vi "State Machine Kernel.vi"(4 "Init?":bool, 5 "Inputs":T4 {"Kobuki Sensors"."Charger Source" items=["DISCHARGING"=0, "DOCKING_CHARGED"=2, "DOCKING_CHARGING"=6, "ADAPTER_CHARGED"=18, "ADAPTER_CHARGING"=22]; "accelerometer"."z axis (g)" format="%.3f"; "accelerometer"."y axis (g)" format="%.3f"; "accelerometer"."x axis (g)" format="%.3f"}, 7 "StateData In":T1) -> (0 "Terminated?":bool, 2 "Outputs":T3, 3 "StateData Out":T1)   [LabVIEW 2017]
uses:
  controls/Inputs.ctl
  shared/Accelerometer.ctl
  Kobuki/KobukiSensors.ctl
  Kobuki/Kobuki Bumps and WheelDrops.ctl
  Kobuki/Kobuki Buttons.ctl
  controls/Outputs.ctl
  controls/StateData.ctl
  controls/StatesEnum.ctl
panel:
  # "Electrical: charging, battery, OI mode"
  # "Sensors: bump, cliff, button, wheel drop"
  # "Motors:"
  # "Inertia"
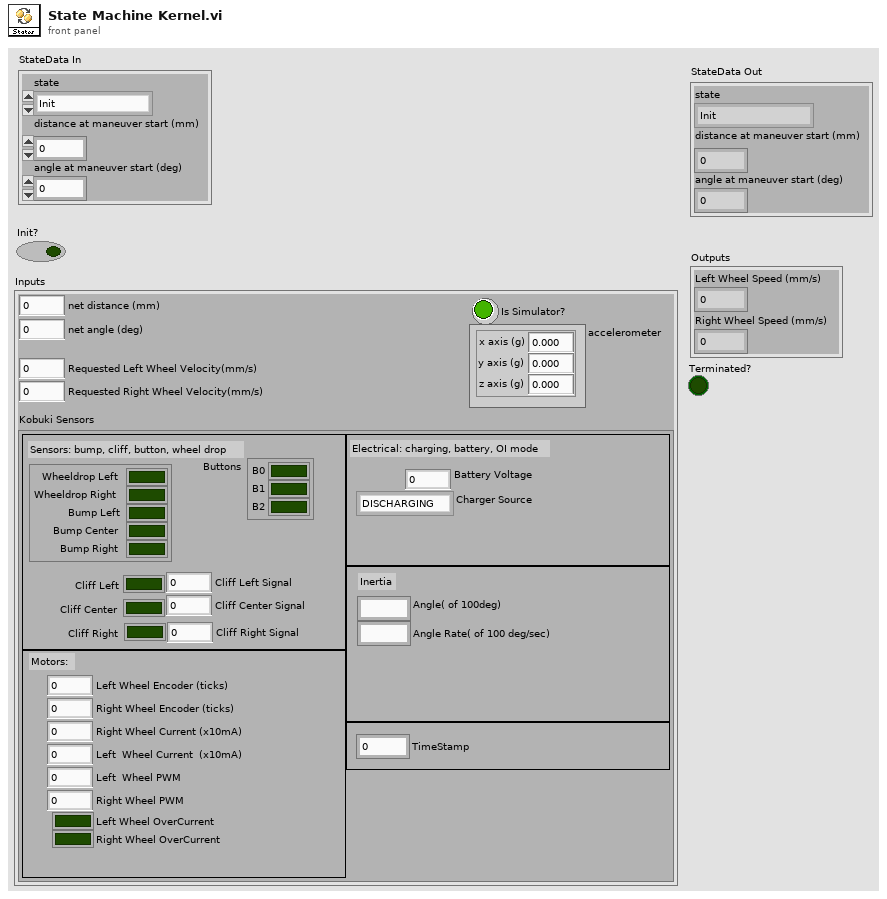
[diagram p1: front panel]
types:
  T1 = typedef "StateData.ctl" = cluster{"distance at maneuver start (mm)":i32, "angle at maneuver start (deg)":i32, "state":T2}
  T2 = typedef "StatesEnum.ctl" = enum16{"Init", "Pause", "Drive", "L.Cliff", "R.Cliff", "Shut"}
  T3 = typedef "Outputs.ctl" = cluster{"Left Wheel Speed (mm/s)":i16, "Right Wheel Speed (mm/s)":i16}
  T4 = typedef "Inputs.ctl" = cluster{"net distance (mm)":i32, "net angle (deg)":i32, "accelerometer":T5, "Is Simulator?":bool, "Kobuki Sensors":T6, "Requested Left Wheel Velocity(mm/s)":i32, "Requested Right Wheel Velocity(mm/s)":i32}
  T5 = typedef "Accelerometer.ctl" = cluster{"x axis (g)":dbl, "y axis (g)":dbl, "z axis (g)":dbl}
  T6 = typedef "KobukiSensors.ctl" = cluster{"Bumps + Wheel Drops":T7, "Cliff Left":bool, "Cliff Center":bool, "Cliff Right":bool, "Cliff Left Signal":u16, "Cliff Center Signal":u16, "Cliff Right Signal":u16, "Buttons":T8, "Left Wheel Encoder (ticks)":u16, "Right Wheel Encoder (ticks) ":u16, "Left  Wheel PWM":i8, "Right Wheel PWM":i8, "Left Wheel OverCurrent":bool, "Right Wheel OverCurrent ":bool, "Right Wheel Current (x10mA)":i16, "Left  Wheel Current  (x10mA)":i16, "TimeStamp":u16, "Battery Voltage":dbl, "Angle( of 100deg)":i16, "Angle Rate( of 100 deg/sec)":i16, "Charger Source ":i8}
  T7 = typedef "Kobuki Bumps and WheelDrops.ctl" = cluster{"Wheeldrop Left":bool, "Wheeldrop Right":bool, "Bump Left":bool, "Bump Center":bool, "Bump Right":bool}
  T8 = typedef "Kobuki Buttons.ctl" = cluster{"B0":bool, "B1":bool, "B2":bool}
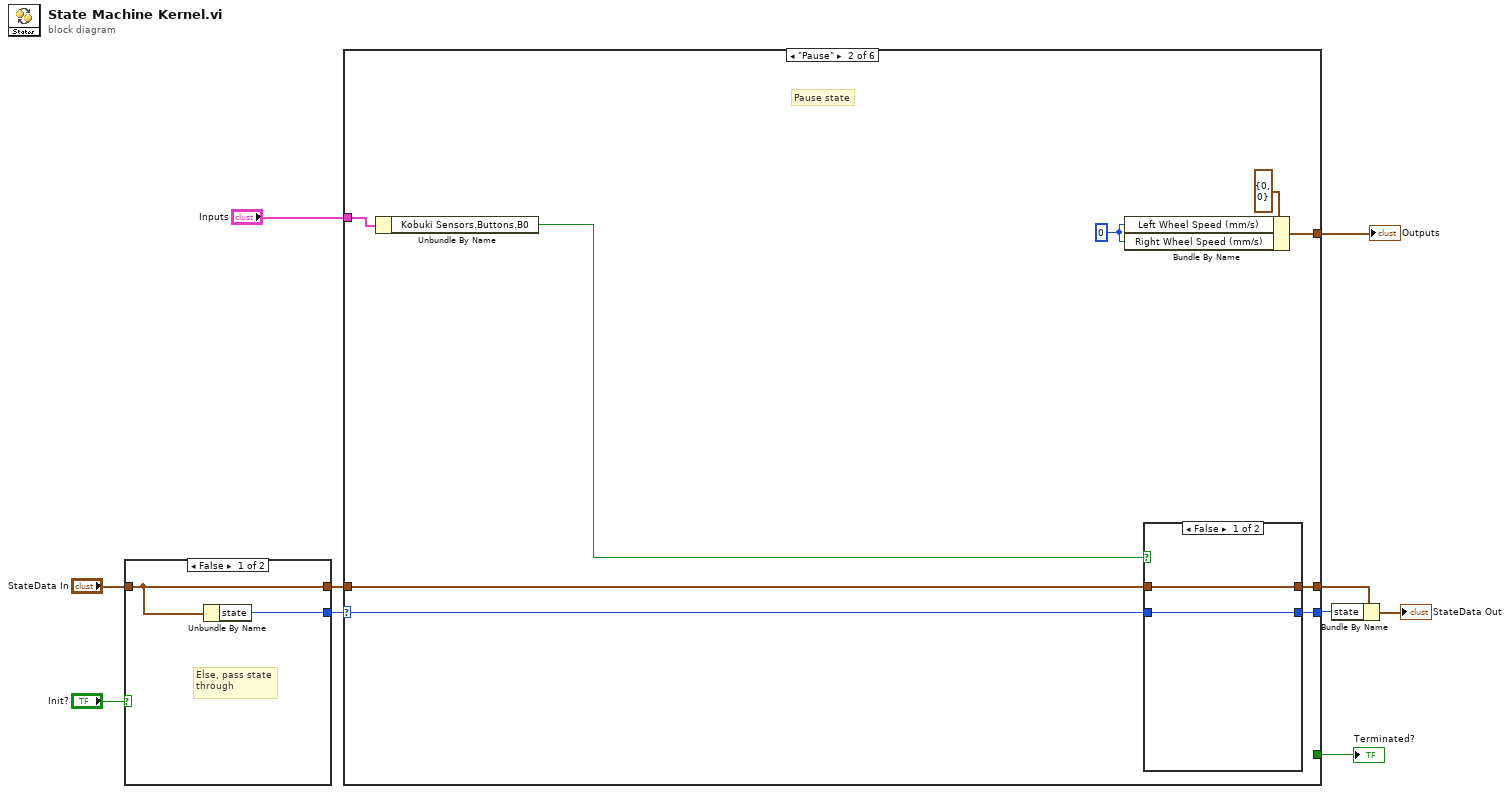
[diagram p0: block diagram]
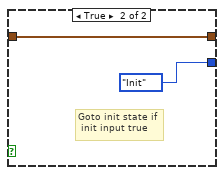
[diagram p2: hidden frame]
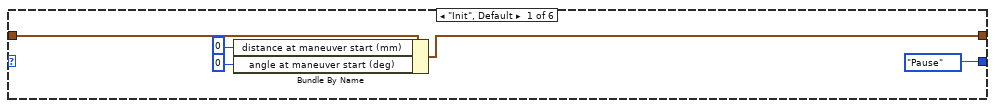
[diagram p3: hidden frame]
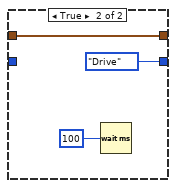
[diagram p4: hidden frame]
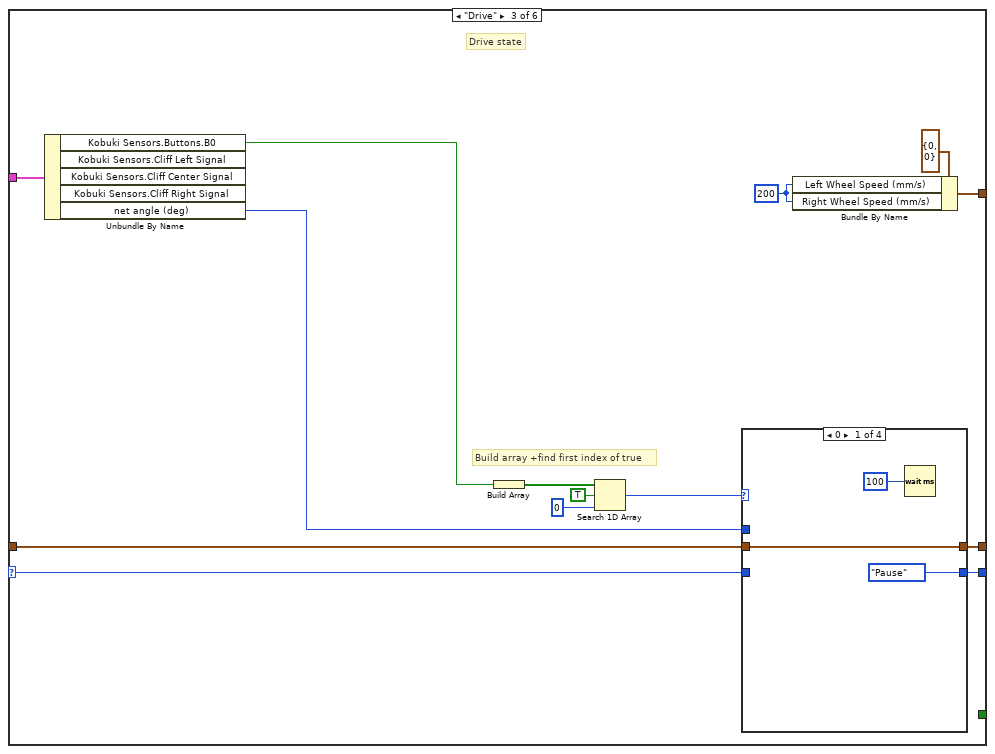
[diagram p5: hidden frame]
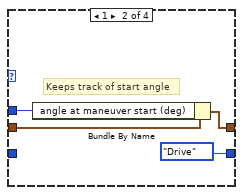
[diagram p6: hidden frame]
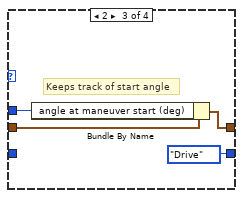
[diagram p7: hidden frame]
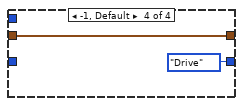
[diagram p8: hidden frame]
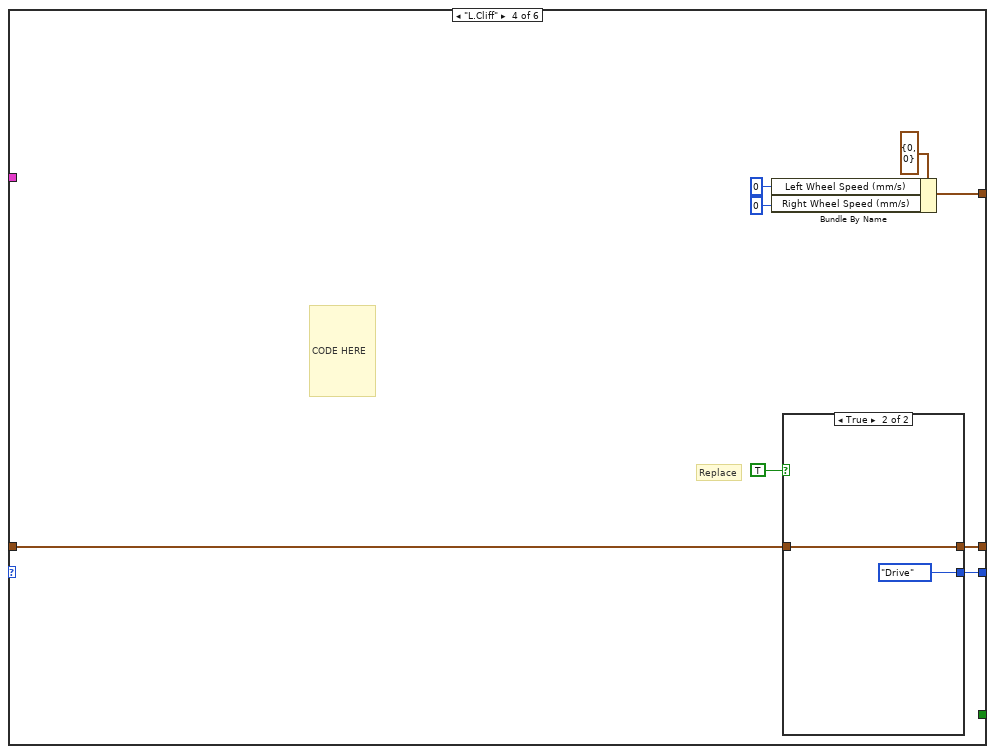
[diagram p9: hidden frame]
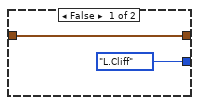
[diagram p10: hidden frame]
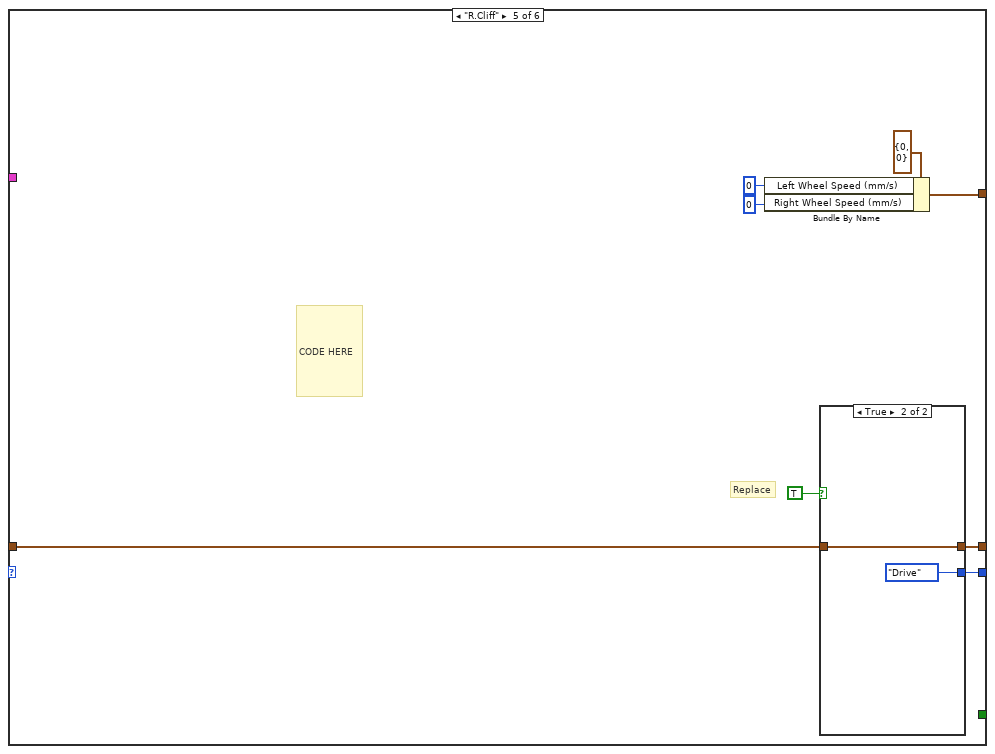
[diagram p11: hidden frame]
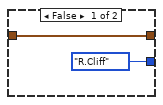
[diagram p12: hidden frame]
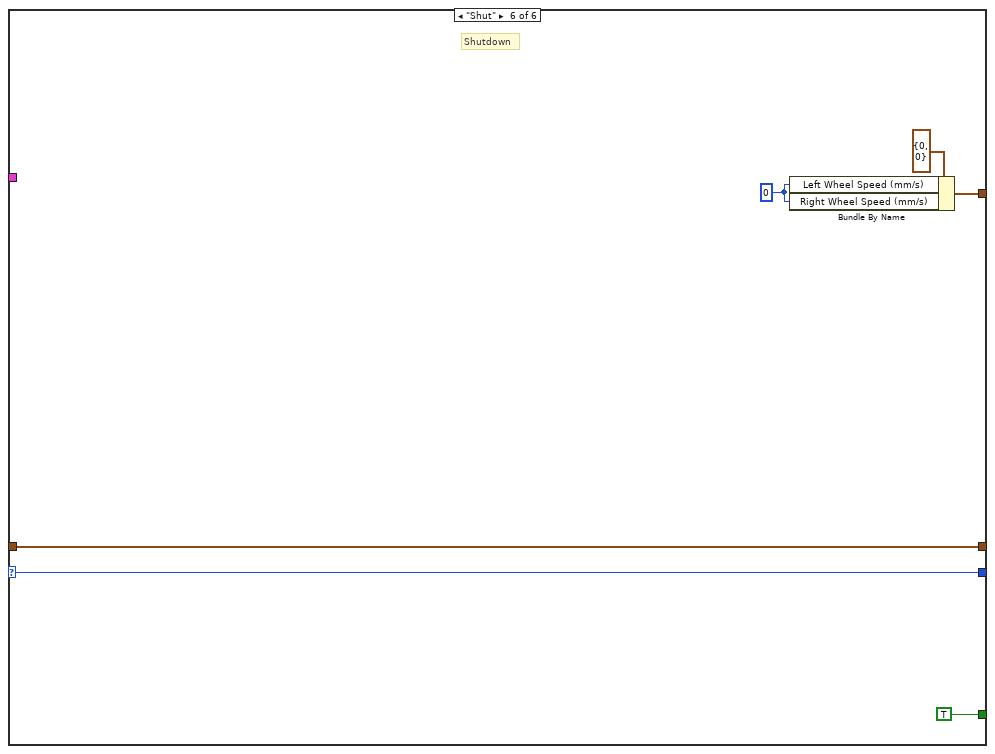
[diagram p13: hidden frame]
diagram:
  n1 = case shown="False" "Init?" {
    tunnel: [w12 StatesEnum."Init" ("StateIn")] -> w8
    tunnel: "StateData In" -> [w11 w13]
    tunnel: [w11 w13] -> w3
    frame False {
      # "Else, pass state \nthrough"
      n2 = Unbundle By Name(w11) -> ("state"=w12:T2)
    }
    frame True {
      # "Goto init state if\n init input true"
    }
  }
  n3 = case shown="\"Pause\"" w8 {
    selector: w8 -> [_ w24 w46 _ _ w90]
    tunnel: [StatesEnum."Pause" ("StateIn") w23 w45 w66 w77 w90] -> w5
    tunnel: "Inputs" -> [_ w25 w47 _ _ _]
    tunnel: [_ w28 w43 w67 w76 w87] -> w6
    tunnel: [_ _ _ _ _ TRUE] -> w7
    tunnel: w3 -> [w18 w21 w36 w62 w74 w85]
    tunnel: [w17 w20 w35 w63 w75 w85] -> w2
    frame "Init", Default {
      n4 = Bundle By Name(cluster=w18, "distance at maneuver start (mm)"=0, "angle at maneuver start (deg)"=0) -> (w17:T1)
    }
    frame "Pause" {
      w27 = i16 0 ("Left Wheel Speed (mm/s)")
      # "Pause state"
      n5 = Unbundle By Name(w25) -> ("Kobuki Sensors.Buttons.B0"=w26:bool)
      n6 = Bundle By Name(cluster=T3 {"Left Wheel Speed (mm/s)"=0, "Right Wheel Speed (mm/s)"=0} ("Outputs"), "Left Wheel Speed (mm/s)"=w27, "Right Wheel Speed (mm/s)"=w27) -> (w28:T3)
      n7 = case shown="False" w26 {
        tunnel: w24 -> [w30 _]
        tunnel: [w30 StatesEnum."Drive" ("StateIn")] -> w23
        tunnel: w21 -> [w29 w31]
        tunnel: [w29 w31] -> w20
        frame False {
        }
        frame True {
          n8 = Wait (ms)(milliseconds to wait=u32 100) -> ()  [unwired: 1 out]
        }
      }
    }
    frame "Drive" {
      w42 = i16 200
      # "Build array +find first index of true"
      # "Drive state"
      n9 = Unbundle By Name(w47) -> ("Kobuki Sensors.Buttons.B0"=w41:bool, "net angle (deg)"=w34:i32)  [unwired: 3 out]
      n10 = Build Array(w41) -> (w40:bool[])
      n11 = Search 1D Array(1D array=w40, element=TRUE, start index (0)=0) -> (index of element=w37:i32)
      n12 = case shown="0" w37 {
        tunnel: w46 -> [_ _ _ _]
        tunnel: [StatesEnum."Pause" ("StateIn") StatesEnum."Drive" ("StateIn") StatesEnum."Drive" ("StateIn") StatesEnum."Drive" ("StateIn")] -> w45
        tunnel: w36 -> [w48 w53 w57 w59]
        tunnel: [w48 w51 w56 w59] -> w35
        tunnel: w34 -> [_ w52 w55 _]
        frame 0 {
          n13 = Wait (ms)(milliseconds to wait=u32 100) -> ()  [unwired: 1 out]
        }
        frame 1 {
          # "Keeps track of start angle"
          n14 = Bundle By Name(cluster=w53, "angle at maneuver start (deg)"=w52) -> (w51:T1)
        }
        frame 2 {
          # "Keeps track of start angle"
          n15 = Bundle By Name(cluster=w57, "angle at maneuver start (deg)"=w55) -> (w56:T1)
        }
        frame -1, Default {
        }
      }
      n16 = Bundle By Name(cluster=T3 {"Left Wheel Speed (mm/s)"=0, "Right Wheel Speed (mm/s)"=0} ("Outputs"), "Left Wheel Speed (mm/s)"=w42, "Right Wheel Speed (mm/s)"=w42) -> (w43:T3)
    }
    frame "L.Cliff" {
      # "Replace"
      # "CODE HERE"
      n17 = Bundle By Name(cluster=T3 {"Left Wheel Speed (mm/s)"=0, "Right Wheel Speed (mm/s)"=0} ("Outputs"), "Left Wheel Speed (mm/s)"=i16 0, "Right Wheel Speed (mm/s)"=i16 0) -> (w67:T3)
      n18 = case shown="True" TRUE {
        tunnel: [StatesEnum."L.Cliff" ("StateIn") StatesEnum."Drive" ("StateIn")] -> w66
        tunnel: w62 -> [w69 w71]
        tunnel: [w69 w71] -> w63
        frame False {
        }
        frame True {
        }
      }
    }
    frame "R.Cliff" {
      # "Replace"
      # "CODE HERE"
      n19 = Bundle By Name(cluster=T3 {"Left Wheel Speed (mm/s)"=0, "Right Wheel Speed (mm/s)"=0} ("Outputs"), "Left Wheel Speed (mm/s)"=i16 0, "Right Wheel Speed (mm/s)"=i16 0) -> (w76:T3)
      n20 = case shown="True" TRUE {
        tunnel: [StatesEnum."R.Cliff" ("StateIn") StatesEnum."Drive" ("StateIn")] -> w77
        tunnel: w74 -> [w81 w83]
        tunnel: [w81 w83] -> w75
        frame False {
        }
        frame True {
        }
      }
    }
    frame "Shut" {
      w88 = i16 0 ("Left Wheel Speed (mm/s)")
      # "Shutdown"
      n21 = Bundle By Name(cluster=T3 {"Left Wheel Speed (mm/s)"=0, "Right Wheel Speed (mm/s)"=0} ("Outputs"), "Left Wheel Speed (mm/s)"=w88, "Right Wheel Speed (mm/s)"=w88) -> (w87:T3)
    }
  }
  "Terminated?" <- w7
  "Outputs" <- w6
  n22 = Bundle By Name(cluster=w2, "state"=w5) -> (→"StateData Out":T1)
